vi "Keithley 2450 Setup and Read Volt.vi"(8 "Error In":errorcluster, 11 "VISA Refnum in":refnum<visa-resource-name>) -> (0 "Error Out":errorcluster, 2 "Voltage":dbl format="%_6g", 3 "VISA Refnum out":refnum<visa-resource-name>)   [LabVIEW 2021]
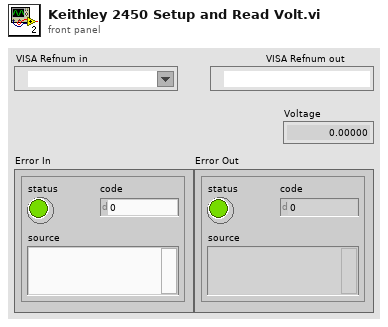
[diagram p1: front panel]
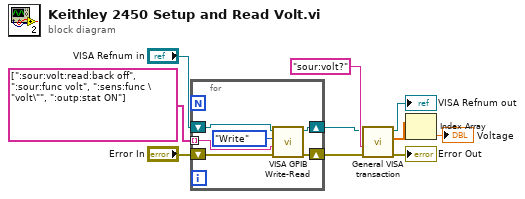
[diagram p0: block diagram]
diagram:
  n1 = for {
    tunnel: string[] [":sour:volt:read:back off", ":sour:func volt", ":sens:func \"volt\"", ":outp:stat ON"] -> [w15] mode=indexing
    shift-right: [w13] -> w5
    shift-left: "Error In" -> [w14]
    shift-right: [w12] -> w3
    shift-left: "VISA Refnum in" -> [w11]
    n2 = call "VISA GPIB Write-Read.vi"("error in (no error)"=w14, "Command"=w15, "Action"=enum16{"Write", "Read", "Write & Read"}."Write", "VISA resource name"=w11) -> ("error out"=w13:errorcluster, "dup VISA Session"=w12:refnum<visa-resource-name>)  [unwired: 4 in, 2 out]
  }
  n3 = call "General VISA transaction.vi"("error in (no error)"=w5, "Command String"="sour:volt?", "VISA Session"=w3) -> ("error out"=→"Error Out":errorcluster, "Measurement"=w9:dbl[], "dup VISA Session"=→"VISA Refnum out":refnum<visa-resource-name>)  [unwired: 3 in, 3 out]
  n4 = Index Array(array=w9) -> (element=→"Voltage":dbl)  [unwired: 1 in]
